vi "19.6-Cascade-4th Order.vi"() -> ()   [LabVIEW 2020]
doc: "Uses the Median Filter VI to analyze pulses in the presence of noise. The example generates a pulse contaminated with Gaussian noise and applies a median filter. For comparison purposes, the VI computes the pulse parameters of the filtered pulse."
uses:
  <vilib>/Analysis/3filter.llb/IIR Filter (DBL).vi
  <vilib>/Analysis/baseanly.llb/IIR Cascade Filter (DBL).vi
  <vilib>/Analysis/NI_AALBase.lvlib
panel:
  out "Single":dbl[](graph)
  out "4th-C2-LV":dbl[](graph)
  out "4th-C2":dbl[](graph)
  out "2nd-D":dbl[](graph)
  in  "Signal":u16(ring) items=["Impulse", "Step"]
  in  "stop":bool
  out "Signal":dbl[](graph)
  in  "Fc":dbl(slide)=299.22077922077926 step=1.0 scale=1.0..512.0 scale format="%#_2f"
  out "2nd-C":dbl[](graph)
  out "4th-C1":dbl[](graph)
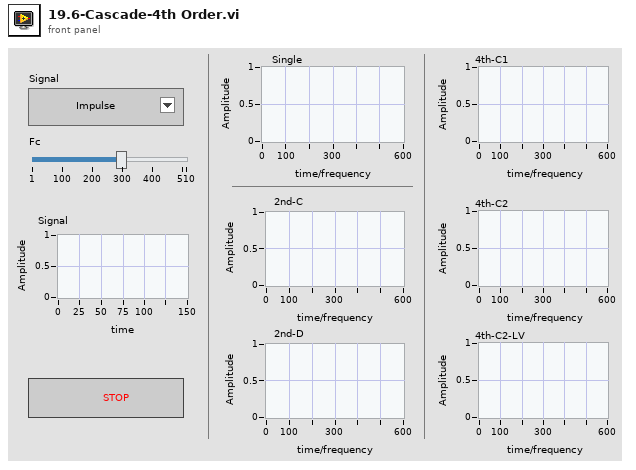
[diagram p1: front panel]
types:
  T1 = cluster{"filter structure":enum32{"IIR 2nd Order", "IIR 4th Order"}, "Reverse Coefficients":dbl[], "Forward Coefficients":dbl[]}
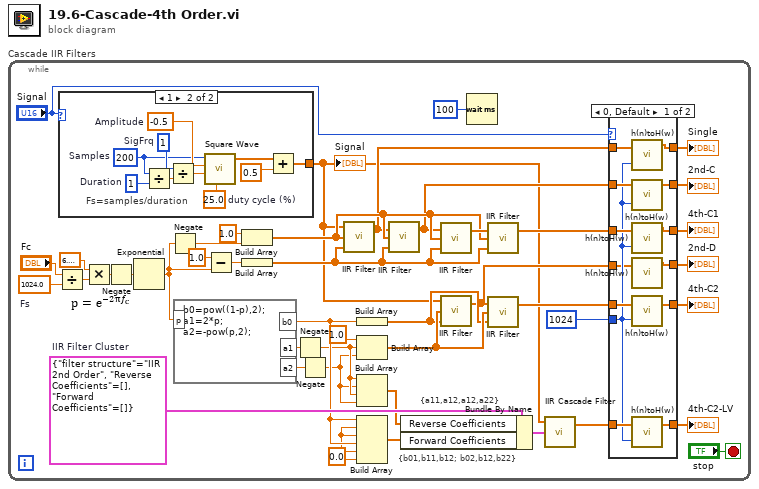
[diagram p0: block diagram]
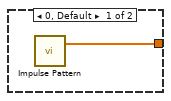
[diagram p3: hidden frame]
diagram:
  n1 = while "Cascade IIR Filters" {
    stop <- "stop" stop-if-true
    w19 = 0.0 ("element")
    w36 = T1 {"filter structure"=enum."IIR 2nd Order", "Reverse Coefficients"=[], "Forward Coefficients"=[]}  # IIR Filter Cluster
    w37 = 1024.0  # Fs
    # "{a11,a12,a12,a22}"
    # "{b01,b11,b12; b02,b12,b22}"
    n2 = Divide(x="Fc", y=w37) -> (x/y=w42:dbl)
    n3 = case shown="1" "Signal" {
      tunnel: [w64 w65] -> w1
      frame 0, Default {
        n4 = call <vilib>:"Impulse Pattern.vi"() -> ("Impulse Pattern"=w64:dbl[])  [unwired: 3 in, 1 out]
      }
      frame 1 {
        w66 = 1  # Duration
        w72 = 1  # SigFrq
        w73 = 25.0  # duty cycle (%)
        w74 = -0.5  # Amplitude
        w68 = 200  # Samples
        # "Fs=samples/duration"
        n5 = Divide(x=w68, y=w66) -> (x/y=w67:dbl)
        n6 = Divide(x=w72, y=w67) -> (x/y=w69:dbl)
        n7 = call <vilib>:"Square Wave.vi"("samples"=w68, "amplitude"=w74, "frequency"=w69, "duty cycle (%)"=w73) -> ("square wave"=w71:dbl[])  [unwired: 2 in, 2 out]
        n8 = Add(x=w71, y=0.5) -> (x+y=w65:dbl[])
      }
    }
    "Signal" <- w1
    n9 = Multiply(x=6.283185307179586, y=w42) -> (x*y=w40:dbl)
    n10 = Negate(x=w40) -> (-x=w41:dbl)
    n11 = Exponential(1:w41) -> (0:w24:dbl)
    n12 = Negate(x=w24) -> (-x=w32:dbl)
    n13 = formula code="b0=pow((1-p),2);\na1=2*p;\na2=-pow(p,2);"("p"=w24) -> ("b0"=w23:dbl, "a1"=w26:dbl, "a2"=w27:dbl)
    n14 = Subtract(x=1.0, y=w24) -> (x-y=w31:dbl)
    n15 = Build Array(1.0 ("element"), w32) -> (w28:dbl[])
    n16 = Build Array(w31) -> (w29:dbl[])
    n17 = Negate(x=w26) -> (-x=w22:dbl)
    n18 = Negate(x=w27) -> (-x=w21:dbl)
    n19 = call-poly <vilib>:"IIR Filter.vi"("Forward Coefficients"=w29, "Reverse Coefficients"=w28, "X"=w1) -> ("Filtered X"=w11:dbl[])  [unwired: 1 in, 1 out]
    n20 = Build Array(w23) -> (w16:dbl[])
    n21 = Build Array(1.0 ("element"), w22, w21) -> (w17:dbl[])
    n22 = Build Array(w22, w21, w22, w21) -> (w20:dbl[])
    n23 = Build Array(w23, w19, w19, w23, w19, w19) -> (w35:dbl[])
    n24 = call-poly <vilib>:"IIR Filter.vi"("Forward Coefficients"=w29, "Reverse Coefficients"=w28, "X"=w11) -> ("Filtered X"=w10:dbl[])  [unwired: 1 in, 1 out]
    n25 = Bundle By Name(cluster=w36, "Reverse Coefficients"=w20, "Forward Coefficients"=w35) -> (w18:T1)
    n26 = call-poly <vilib>:"IIR Filter.vi"("Forward Coefficients"=w29, "Reverse Coefficients"=w28, "X"=w10) -> ("Filtered X"=w30:dbl[])  [unwired: 1 in, 1 out]
    n27 = call-poly <vilib>:"IIR Filter.vi"("Forward Coefficients"=w16, "Reverse Coefficients"=w17, "X"=w1) -> ("Filtered X"=w9:dbl[])  [unwired: 1 in, 1 out]
    n28 = Wait (ms)(milliseconds to wait=u32 100) -> ()  [unwired: 1 out]
    n29 = call-poly <vilib>:"IIR Filter.vi"("Forward Coefficients"=w29, "Reverse Coefficients"=w28, "X"=w30) -> ("Filtered X"=w15:dbl[])  [unwired: 1 in, 1 out]
    n30 = call-poly <vilib>:"IIR Filter.vi"("Forward Coefficients"=w16, "Reverse Coefficients"=w17, "X"=w9) -> ("Filtered X"=w14:dbl[])  [unwired: 1 in, 1 out]
    n31 = call-poly <vilib>:"IIR Cascade Filter.vi"("IIR Filter Cluster"=w18, "X"=w1) -> ("Filtered X"=w13:dbl[])  [unwired: 1 in, 1 out]
    n32 = case shown="0, Default" "Signal" {
      tunnel: w15 -> [w57 w63]
      tunnel: w14 -> [w56 w62]
      tunnel: w13 -> [w55 w61]
      tunnel: [w54 w63] -> w6
      tunnel: [w53 w62] -> w4
      tunnel: [w52 w61] -> w3
      tunnel: w11 -> [w50 w60]
      tunnel: w10 -> [w49 w59]
      tunnel: w9 -> [w46 w58]
      tunnel: [w51 w60] -> w2
      tunnel: [w48 w59] -> w8
      tunnel: 1024 ("FFT size") -> [w47 _]
      tunnel: [w45 w58] -> w5
      frame 0, Default {
        n33 = call "h(n)toH(w).vi"("h(n)"=w50, "FFT size"=w47) -> ("Mag H(w)"=w51:dbl[])  [unwired: 2 out]
        n34 = call "h(n)toH(w).vi"("h(n)"=w49, "FFT size"=w47) -> ("Mag H(w)"=w48:dbl[])  [unwired: 2 out]
        n35 = call "h(n)toH(w).vi"("h(n)"=w57, "FFT size"=w47) -> ("Mag H(w)"=w54:dbl[])  [unwired: 2 out]
        n36 = call "h(n)toH(w).vi"("h(n)"=w46) -> ("Mag H(w)"=w45:dbl[])  [unwired: 1 in, 2 out]
        n37 = call "h(n)toH(w).vi"("h(n)"=w56, "FFT size"=w47) -> ("Mag H(w)"=w53:dbl[])  [unwired: 2 out]
        n38 = call "h(n)toH(w).vi"("h(n)"=w55, "FFT size"=w47) -> ("Mag H(w)"=w52:dbl[])  [unwired: 2 out]
      }
      frame 1 {
      }
    }
    "4th-C1" <- w6
    "2nd-C" <- w8
    "2nd-D" <- w5
    "4th-C2" <- w4
    "4th-C2-LV" <- w3
    "Single" <- w2
  }
